vi "PV error_handling.vi"(7 "Data Typ in":string, 8 "error in":errorcluster, 9 "response (data) in":string, 10 "Parameter\nread only<->describe":bool, 11 "data in":string) -> (0 "error out":errorcluster, 2 "Data out":string, 3 "PV Protocol Data out":string)   [LabVIEW 2024, in "Pfeiffer Vacuum.lvlib"]
uses:
  <instrlib>/Pfeiffer Vacuum/Pfeiffer Vacuum.lvlib
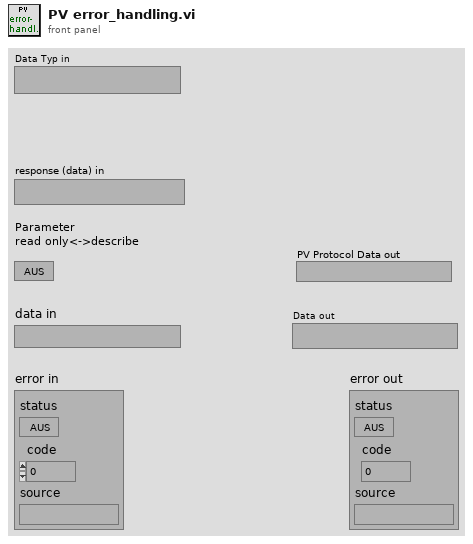
[diagram p1: front panel]
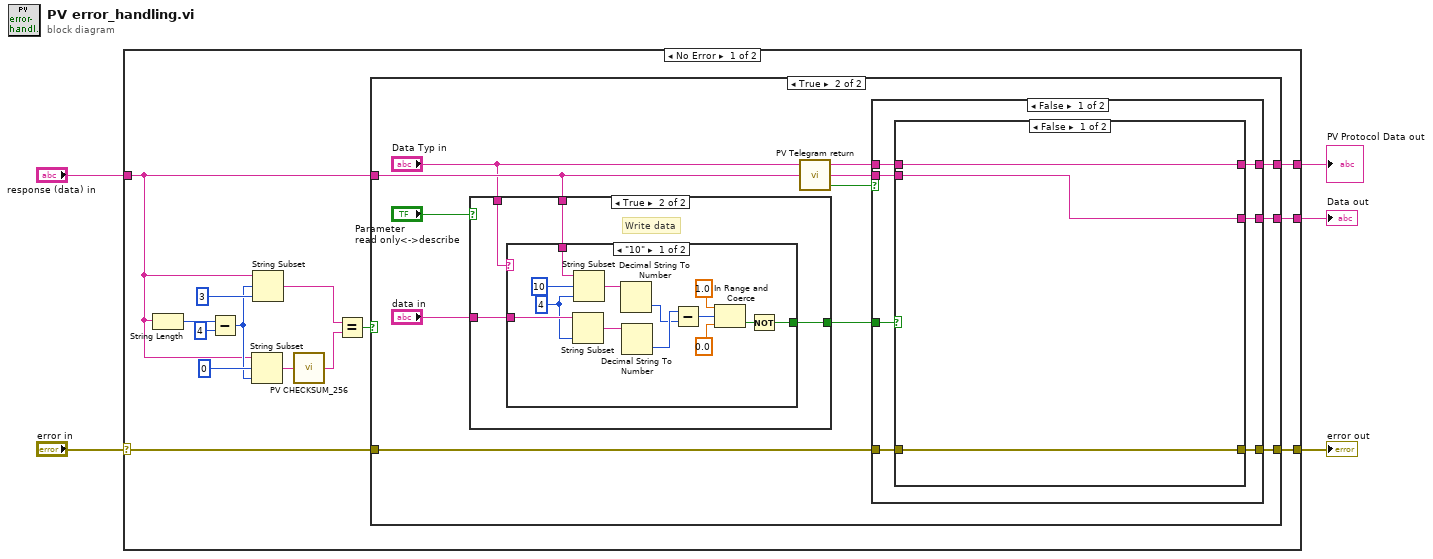
[diagram p0: block diagram]
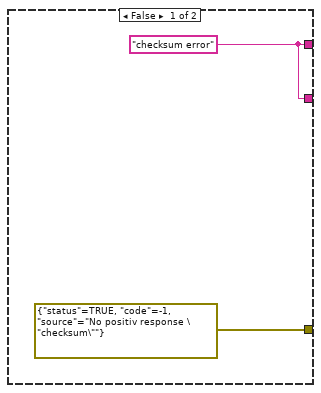
[diagram p2: hidden frame]
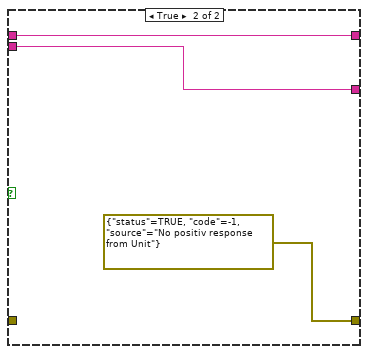
[diagram p3: hidden frame]
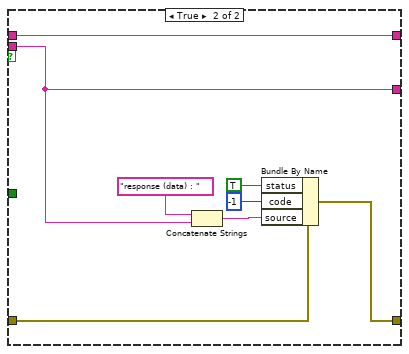
[diagram p4: hidden frame]
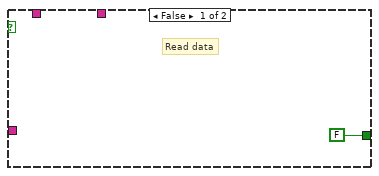
[diagram p5: hidden frame]
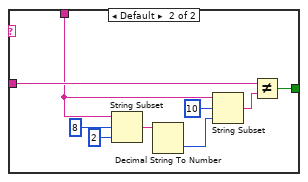
[diagram p6: hidden frame]
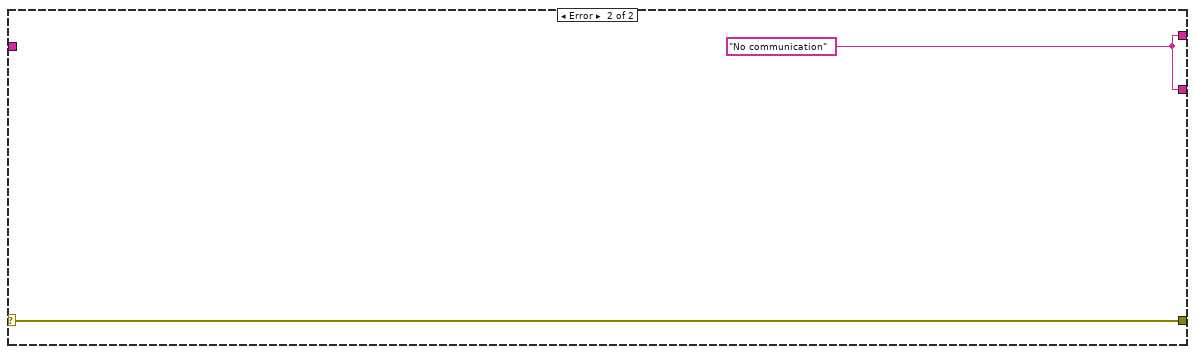
[diagram p7: hidden frame]
diagram:
  n1 = case shown="No Error" "error in" {
    selector: "error in" -> [w7 w83]
    tunnel: [w19 w83] -> w2
    tunnel: "response (data) in" -> [w10 _]
    tunnel: [w8 w82] -> w4
    tunnel: [w6 w82] -> w3
    frame No Error {
      n2 = String Length(string=w10) -> (length=w16:i32)
      n3 = Subtract(x=w16, y=4) -> (x-y=w13:i32)
      n4 = String Subset(string=w10, offset (0)=0 ("Offset (0)"), length (rest)=w13) -> (substring=w12:string)
      n5 = String Subset(string=w10, offset (0)=w13, length (rest)=3 ("Länge (Rest)")) -> (substring=w18:string)
      n6 = call <instrlib>:"PV CHECKSUM_256.VI"("input string"=w12) -> ("checksum"=w11:string)
      n7 = Equal?(x=w18, y=w11) -> (x = y?=w9:bool)
      n8 = case shown="True" w9 {
        tunnel: [errorcluster {"status"=TRUE, "code"=-1, "source"="No positiv response \"checksum\""} ("Fehlerausgang") w31] -> w19
        tunnel: w10 -> [_ w27]
        tunnel: w7 -> [_ w28]
        tunnel: [w20 w29] -> w8
        tunnel: [w20 w25] -> w6
        frame False {
          w20 = "checksum error" ("source")
        }
        frame True {
          n9 = case shown="True" "Parameter\nread only<->describe" {
            tunnel: "data in" -> [_ w59]
            tunnel: [FALSE w58] -> w32
            tunnel: w27 -> [_ w57]
            tunnel: "Data Typ in" -> [_ w56]
            frame False {
              # "Read data"
              # "read data"
            }
            frame True {
              # "Write data"
              # "write date"
              n10 = case shown="\"10\"" w56 {
                tunnel: w59 -> [w70 w79]
                tunnel: [w60 w78] -> w58
                tunnel: w57 -> [w71 w75]
                frame "10" {
                  w69 = 4 ("Länge (Rest)")
                  n11 = String Subset(string=w70, length (rest)=w69) -> (substring=w67:string)  [unwired: 1 in]
                  n12 = String Subset(string=w71, offset (0)=10 ("Offset (0)"), length (rest)=w69) -> (substring=w68:string)
                  n13 = Decimal String To Number(string=w68) -> (number=w63:i32)  [unwired: 2 in, 1 out]
                  n14 = Decimal String To Number(string=w67) -> (number=w64:i32)  [unwired: 2 in, 1 out]
                  n15 = Subtract(x=w64, y=w63) -> (x-y=w61:i32)
                  n16 = In Range and Coerce(upper limit=1.0 ("x"), x=w61, lower limit=0.0 ("Untergrenze")) -> (In Range?=w65:bool)  [unwired: 1 out]
                  n17 = Not(x=w65) -> (.not. x?=w60:bool)
                }
                frame Default {
                  n18 = String Subset(string=w75, offset (0)=8 ("Offset (0)"), length (rest)=2 ("Länge (Rest)")) -> (substring=w74:string)
                  n19 = Decimal String To Number(string=w74) -> (number=w73:i32)  [unwired: 2 in, 1 out]
                  n20 = String Subset(string=w75, offset (0)=10 ("Offset (0)"), length (rest)=w73) -> (substring=w80:string)
                  n21 = Not Equal?(x=w79, y=w80) -> (x != y?=w78:bool)
                }
              }
            }
          }
          n22 = call <instrlib>:"PV Telegram return.vi"("String received"=w27, "Data Typ String"="Data Typ in") -> ("error"=w30:bool, "Substring"=w22:string, "PV Protocol Data out"=w26:string)  [unwired: 1 in]
          n23 = case shown="False" w30 {
            tunnel: [w40 w54] -> w31
            tunnel: w22 -> [w38 w48]
            tunnel: w32 -> [w39 _]
            tunnel: [w37 w48] -> w29
            tunnel: w28 -> [w36 w49]
            tunnel: w26 -> [w35 w47]
            tunnel: [w34 w47] -> w25
            frame False {
              n24 = case shown="False" w39 {
                tunnel: [w42 errorcluster {"status"=TRUE, "code"=-1, "source"="No positiv response from Unit"} ("Fehlerausgang")] -> w40
                tunnel: w38 -> [w43 w45]
                tunnel: [w43 w45] -> w37
                tunnel: w36 -> [w42 _]
                tunnel: w35 -> [w41 w44]
                tunnel: [w41 w44] -> w34
                frame False {
                }
                frame True {
                }
              }
            }
            frame True {
              n25 = Concatenate Strings("response (data) : " ("Elemente bündeln"), w48) -> (w50:string)
              n26 = Bundle By Name(cluster=w49, "status"=TRUE ("Elemente bündeln"), "code"=-1 ("Elemente bündeln"), "source"=w50) -> (w54:errorcluster)
            }
          }
        }
      }
    }
    frame Error {
      w82 = "No communication" ("y")
    }
  }
  "error out" <- w2
  "Data out" <- w4
  "PV Protocol Data out" <- w3
